vi "Ler dados brutos.vi"() -> ()   [LabVIEW 2016]
panel:
  out "Dados brutos":dbl[][](graph)
  in  "Arquivo":path
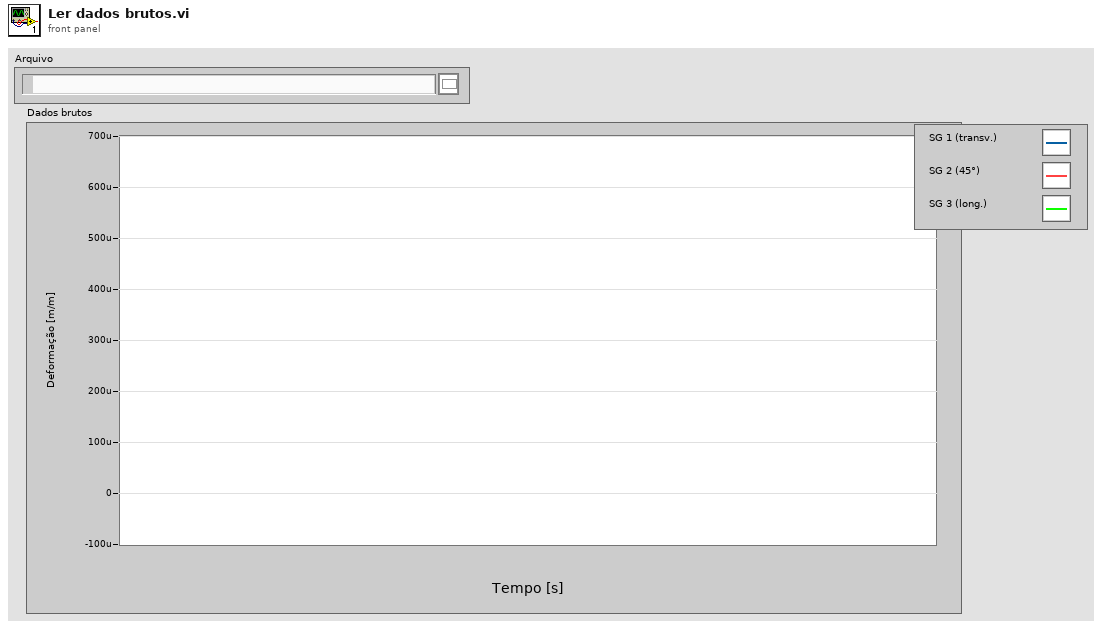
[diagram p1: front panel]
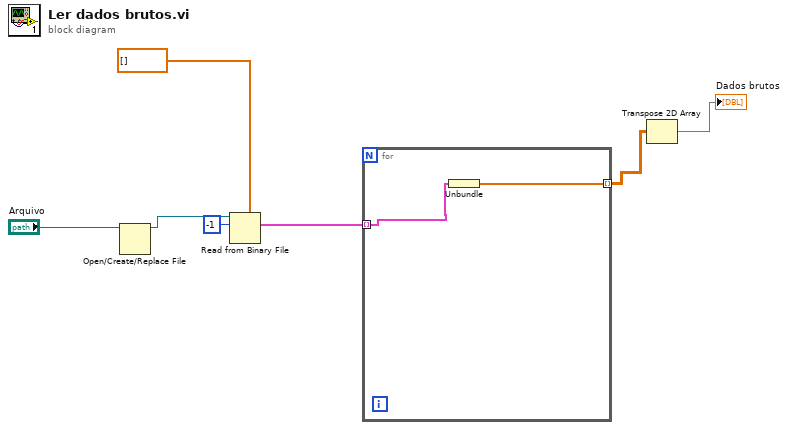
[diagram p0: block diagram]
diagram:
  n1 = Open/Create/Replace File(file path (use dialog)="Arquivo") -> (refnum out=w6:refnum<file>)  [unwired: 5 in, 2 out]
  n2 = Read from Binary File(5:dbl[] [], 10:-1 ("count (1)"), 11:w6) -> (2:w3:cluster{dbl[]}[])  [unwired: 3 in, 3 out]
  n3 = for {
    tunnel: w3 -> [w9] mode=indexing
    tunnel: [w8] -> w2 mode=indexing
    n4 = Unbundle(w9) -> (w8:dbl[])
  }
  n5 = Transpose 2D Array(2D array=w2) -> (transposed array=→"Dados brutos":dbl[][])
